vi "Sweep SL Fine.vi"(8 "error in (no error)":errorcluster, 9 "Sweep outfile":path, 10 "addr":i32, 11 "instrument handle":refnum<k15>) -> (0 "error out":errorcluster, 1 "final current (A)":dbl, 2 "final resistance (ohm)":dbl, 3 "instrument handle out":refnum<k15>)   [LabVIEW 2018]
uses:
  <vilib>/Utility/file.llb/Write Delimited Spreadsheet (DBL).vi
panel:
  out "i":i32
  out "PW":i32
  out "SL voltage (V)":dbl
  out "WL voltage (V)":dbl
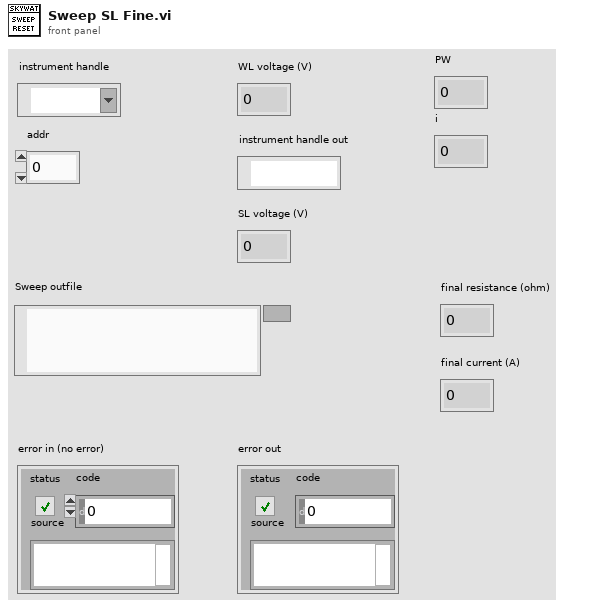
[diagram p1: front panel]
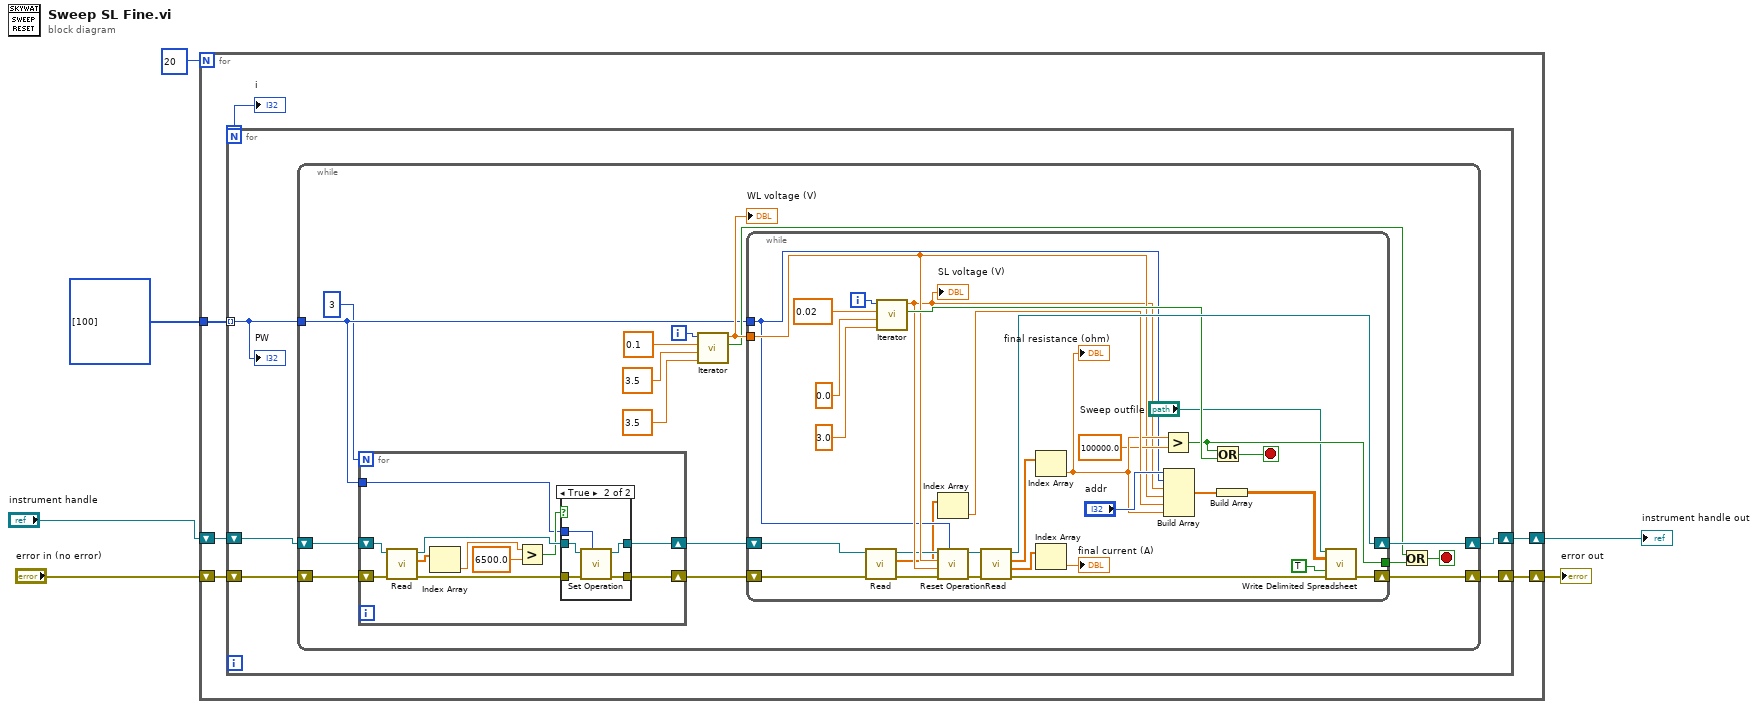
[diagram p0: block diagram]
diagram:
  n1 = for {
    N: 20 -> [_]
    tunnel: i32[] [100] -> [w8]
    shift-right: [w12] -> w6
    shift-left: "instrument handle" -> [w11]
    shift-right: [w9] -> w3
    shift-left: "error in (no error)" -> [w10]
    i -> [w7]
    n2 = for {
      shift-right: [w17] -> w12
      shift-left: w11 -> [w16]
      shift-right: [w14] -> w9
      shift-left: w10 -> [w15]
      tunnel: w8 -> [w13] mode=indexing
      n3 = while {
        shift-right: [w30] -> w17
        shift-left: w16 -> [w23]
        shift-right: [w29] -> w14
        shift-left: w15 -> [w22]
        tunnel: w13 -> [w21]
        i -> [w31]
        stop <- w24 stop-if-true
        n4 = for {
          N: 3 -> [_]
          tunnel: w21 -> [w36]
          shift-right: [w34] -> w19
          shift-left: w23 -> [w38]
          shift-right: [w35] -> w20
          shift-left: w22 -> [w37]
          n5 = call "Read.vi"("error in (no error)"=w37, "instrument handle"=w38) -> ("error out"=w43:errorcluster, "resistances (ohm)"=w39:dbl[], "instrument handle out"=w42:refnum<k15>)  [unwired: 6 in, 1 out]
          n6 = Index Array(array=w39) -> (element=w44:dbl)  [unwired: 1 in]
          n7 = Greater?(x=w44, y=6500.0) -> (0:w41:bool)
          n8 = case shown="True" w41 {
            tunnel: w42 -> [w46 w51]
            tunnel: w43 -> [w45 w50]
            tunnel: [w46 w49] -> w34
            tunnel: [w45 w48] -> w35
            tunnel: w36 -> [_ w47]
            frame False {
            }
            frame True {
              n9 = call "Set Operation.vi"("PW"=w47, "error in (no error)"=w50, "instrument handle"=w51) -> ("error out"=w48:errorcluster, "instrument handle out"=w49:refnum<k15>)  [unwired: 7 in]
            }
          }
        }
        n10 = call "Iterator.vi"("Final Value"=3.5 ("y"), "Initial Value"=3.5 ("y"), "Step"=0.1 ("x"), "i"=w31) -> ("End Loop"=w26:bool, "Current Value"=w27:dbl)  [unwired: 6 in]
        "WL voltage (V)" <- w27
        n11 = while {
          shift-right: [w72] -> w30
          shift-left: w19 -> [w53]
          shift-right: [w75] -> w29
          shift-left: w20 -> [w54]
          tunnel: w27 -> [w60]
          tunnel: w21 -> [w58]
          tunnel: [w63] -> w25
          i -> [w82]
          stop <- w67 stop-if-true
          n12 = call "Read.vi"("error in (no error)"=w54, "instrument handle"=w53) -> ("error out"=w55:errorcluster, "resistances (ohm)"=w52:dbl[], "instrument handle out"=w56:refnum<k15>)  [unwired: 6 in, 1 out]
          n13 = call "Iterator.vi"("Final Value"=3.0 ("y"), "Initial Value"=0.0 ("y"), "Step"=0.02 ("x"), "i"=w82) -> ("End Loop"=w66:bool, "Current Value"=w59:dbl)  [unwired: 6 in]
          "SL voltage (V)" <- w59
          n14 = Index Array(array=w52) -> (element=w68:dbl)  [unwired: 1 in]
          n15 = call "Reset Operation.vi"("PW"=w58, "error in (no error)"=w55, "SLV"=w59, "WLV"=w60, "instrument handle"=w56) -> ("error out"=w62:errorcluster, "instrument handle out"=w61:refnum<k15>)  [unwired: 5 in]
          n16 = call "Read.vi"("error in (no error)"=w62, "instrument handle"=w61) -> ("error out"=w73:errorcluster, "currents (A)"=w70:dbl[], "resistances (ohm)"=w71:dbl[], "instrument handle out"=w72:refnum<k15>)  [unwired: 6 in]
          n17 = Index Array(array=w71) -> (element=w65:dbl)  [unwired: 1 in]
          "final resistance (ohm)" <- w65
          n18 = Index Array(array=w70) -> (element=→"final current (A)":dbl)  [unwired: 1 in]
          n19 = Greater?(x=w65, y=100000.0 ("x")) -> (0:w63:bool)
          n20 = Build Array("addr", w58, w59, w60, w68, w65) -> (w77:dbl[])
          n21 = Or(x=w63, y=w66) -> (x .or. y?=w67:bool)
          n22 = Build Array(w77) -> (w78:dbl[][])
          n23 = call-poly <vilib>:"Write Delimited Spreadsheet.vi"("file path (dialog if empty)"="Sweep outfile", "2D data"=w78, "append to file? (new file:F)"=TRUE, "error in (no error)"=w73) -> ("error out"=w75:errorcluster)  [unwired: 10 in, 1 out]
        }
        n24 = Or(x=w26, y=w25) -> (x .or. y?=w24:bool)
      }
      "PW" <- w13
    }
    "i" <- w7
  }
  "error out" <- w3
  "instrument handle out" <- w6
